vi "_025.vi"(11 "Celsius 2":dbl) -> (3 "Farenheit 2":dbl)   [LabVIEW 2024]
panel:
  out "i++;":dbl
  out "Farenheit":dbl
  in  "Celsius":dbl
  # "Formula Node :"
  # "Celsius -> farenhiet"
  # "( using group of constants )"
  # "Celsius -> farenhiet"
  # "( using FormulaNode )"
  # "increment ;"
  # "The same i/p will assigned to G"
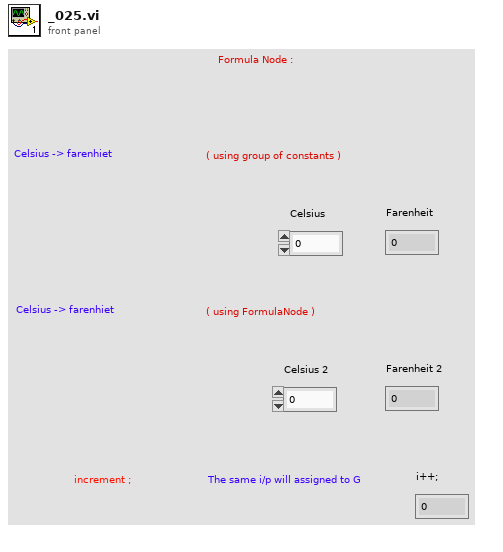
[diagram p1: front panel]
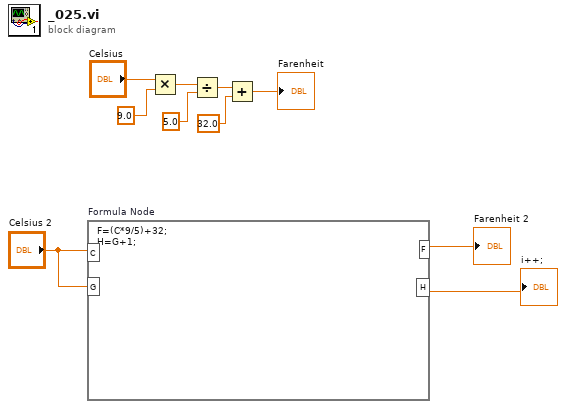
[diagram p0: block diagram]
diagram:
  n1 = formula code="F=(C*9/5)+32;\nH=G+1;"("C"="Celsius 2", "G"="Celsius 2") -> ("F"=→"Farenheit 2":dbl, "H"=→"i++;":dbl)
  n2 = Multiply(x="Celsius", y=9.0) -> (x*y=w8:dbl)
  n3 = Divide(x=w8, y=5.0) -> (x/y=w6:dbl)
  n4 = Add(x=w6, y=32.0) -> (x+y=→"Farenheit":dbl)
